vi "Query Integrate Status.vi"(8 "error in (no error)":errorcluster, 11 "VISA resource name":refnum<visa-resource-name>) -> (0 "error out":errorcluster, 1 "Integrate Status List":bool[](array[boolean]), 2 "Integrate Status":i32, 3 "VISA resource name out":refnum<visa-resource-name>)   [LabVIEW 2016, in "Yokogawa WT300 Series.lvlib"]
doc: "Queries the integration status."
uses:
  Yokogawa WT300 Series.lvlib
panel:
  # "Reset"
  # "Start"
  # "Stop"
  # "Error"
  # "Time up"
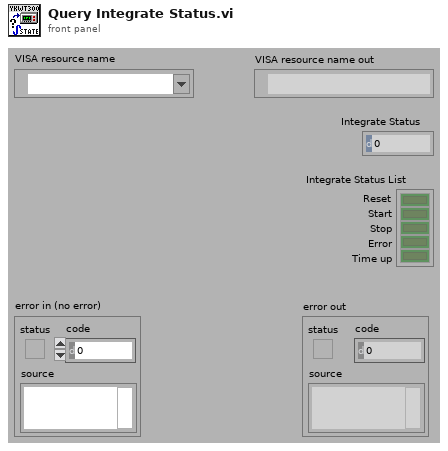
[diagram p1: front panel]
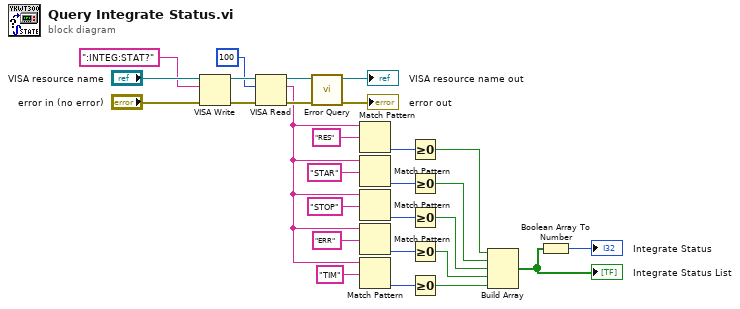
[diagram p0: block diagram]
diagram:
  n1 = VISA Write ("VISA書き込み")(VISA resource name="VISA resource name", write buffer=":INTEG:STAT?" ("Œ`Ž®•¶Žš—ñ"), error in (no error)="error in (no error)") -> (VISA resource name out=w27:refnum<visa-resource-name>, error out=w28:errorcluster)  [unwired: 1 out]
  n2 = VISA Read ("VISA読み取り")(VISA resource name=w27, byte count=u32 100, error in (no error)=w28) -> (VISA resource name out=w25:refnum<visa-resource-name>, read buffer=w16:string, error out=w21:errorcluster)  [unwired: 1 out]
  n3 = call "Error Query.vi"("error in (no error)"=w21, "VISA resource name"=w25) -> ("error out"=→"error out":errorcluster, "VISA resource name out"=→"VISA resource name out":refnum<visa-resource-name>)  [unwired: 6 in, 2 out]
  n4 = Match Pattern(string=w16, regular expression="RES") -> (offset past match=w15:i32)  [unwired: 1 in, 3 out]
  n5 = Match Pattern(string=w16, regular expression="STAR") -> (offset past match=w13:i32)  [unwired: 1 in, 3 out]
  n6 = Match Pattern(string=w16, regular expression="STOP") -> (offset past match=w12:i32)  [unwired: 1 in, 3 out]
  n7 = Match Pattern(string=w16, regular expression="ERR") -> (offset past match=w11:i32)  [unwired: 1 in, 3 out]
  n8 = Match Pattern(string=w16, regular expression="TIM") -> (offset past match=w14:i32)  [unwired: 1 in, 3 out]
  n9 = Greater Or Equal To 0?(x=w15) -> (x >= 0?=w10:bool)
  n10 = Greater Or Equal To 0?(x=w13) -> (x >= 0?=w4:bool)
  n11 = Greater Or Equal To 0?(x=w12) -> (x >= 0?=w3:bool)
  n12 = Greater Or Equal To 0?(x=w11) -> (x >= 0?=w2:bool)
  n13 = Greater Or Equal To 0?(x=w14) -> (x >= 0?=w1:bool)
  n14 = Build Array(w10, w4, w3, w2, w1) -> (w9:bool[])
  "Integrate Status List" <- w9
  n15 = Boolean Array To Number(Boolean array=w9) -> (number=→"Integrate Status":u32)
